vi "tm3samp_framerate_wVision.vi"() -> ()   [LabVIEW 2012]
panel:
  out "Display":T1(plugin-control)
  out "Camera Serial":string
  out "Camera Version":string
  out "Camera Model":string
  out "SMD":dbl
  in  "Scan Mode":dbl min=0.0 max=0.0
  in  "Exposure":dbl min=0.003001263157894737 max=10.0 step=9.74436090225564e-06
  out "EXP":dbl
  out "SVW":i32
  out "SHW":i32
  out "SVO":i32
  out "SHO":i32
  in  "V Width":i32 min=4 max=2048 step=4
  in  "V Offset":i32 min=0 max=0 step=4
  in  "H Width":i32 min=4 max=2048 step=4
  in  "H Offset":i32 min=0 max=0 step=4
  in  "Binning":u16(ring) items=["1x1"=1, "2x2"=2, "4x4"=4]
  out "Elapsed Time":u32
  out "Total Frames":i32
  in  "Display":bool=TRUE
  out "Frames Per Second":dbl
  out "error out":errorcluster
  in  "stop":bool
  # "This example displays the frame rate\nof the camera.  Changing the resolution\nof the camera or displaying the images\nwill affect the frame rate."
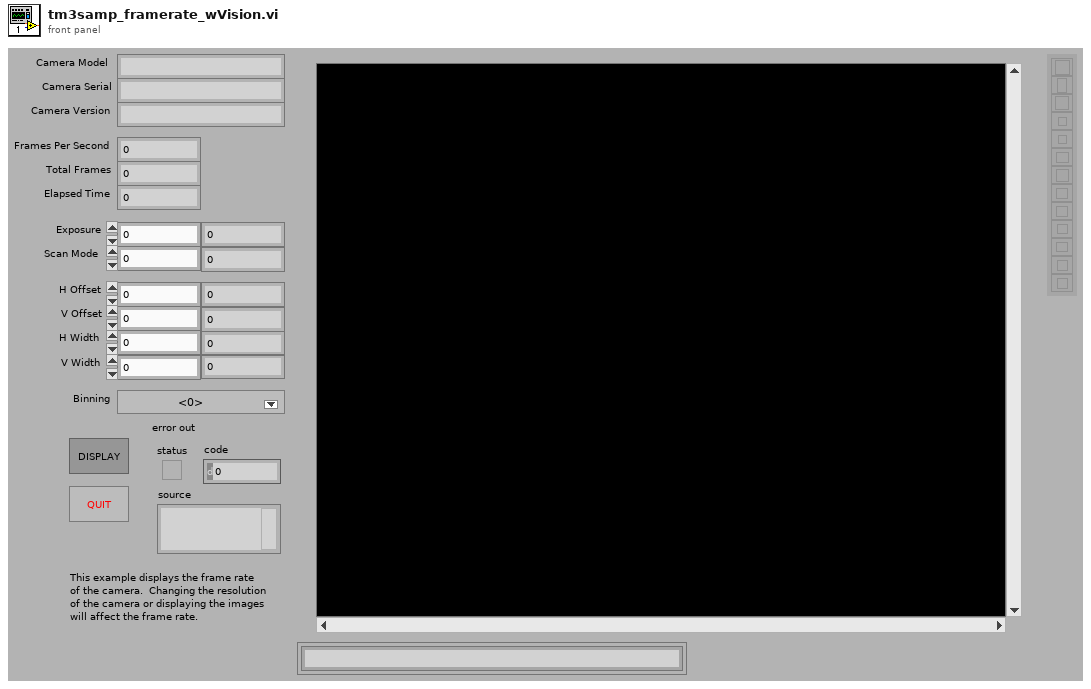
[diagram p1: front panel]
types:
  T1 = typedef "IMAQ Image.ctl" = refnum<image>
  T2 = typedef "Image Type" = u32
  T3 = cluster{"Value":i32, "Minimum":i32, "Maximum":i32, "Increment":i32}
  T4 = cluster{"width":u32, "height":u32, "datatype":u32}
  T5 = cluster{"H Offset":i32, "V Offset":i32, "H Width":i32, "V Width":i32}
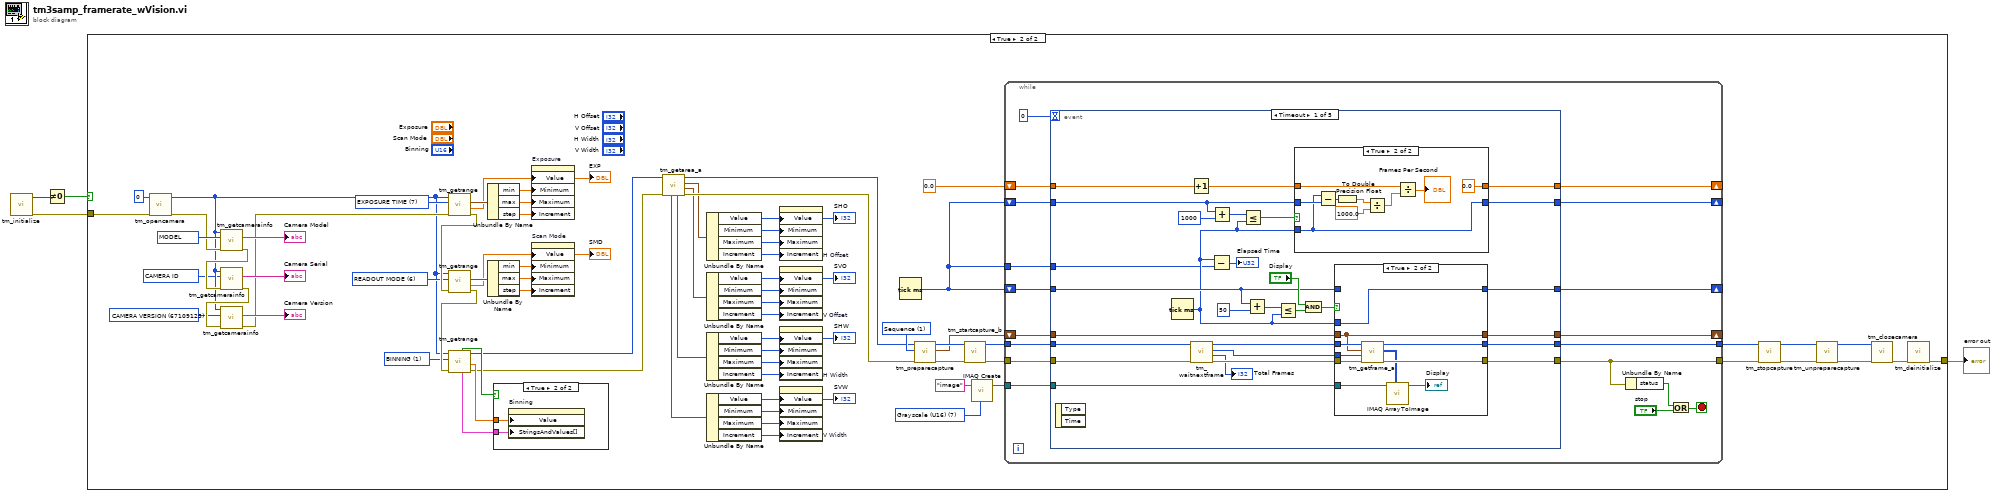
[diagram p0: block diagram]
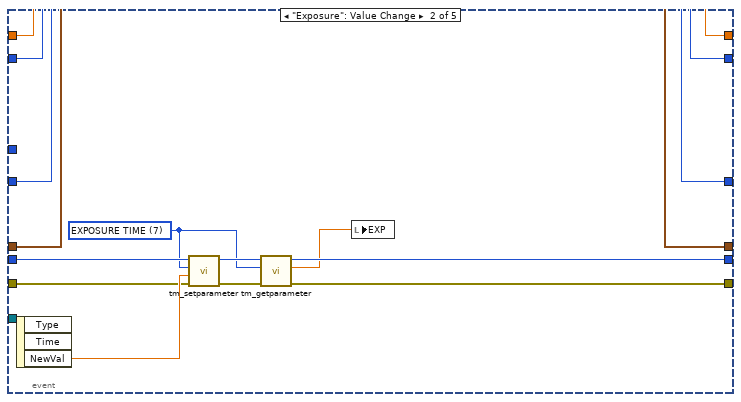
[diagram p6: hidden frame]
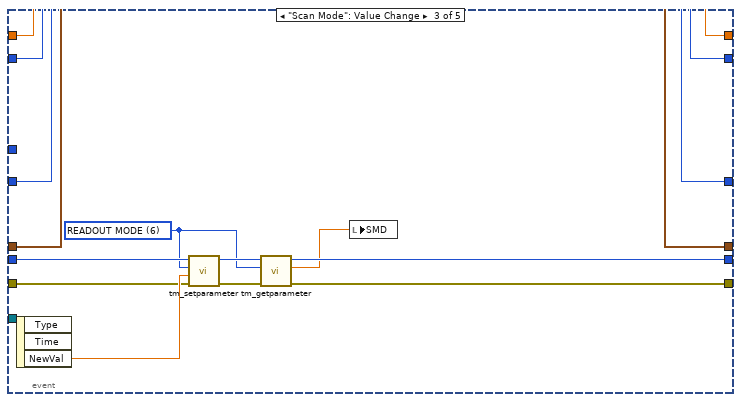
[diagram p7: hidden frame]
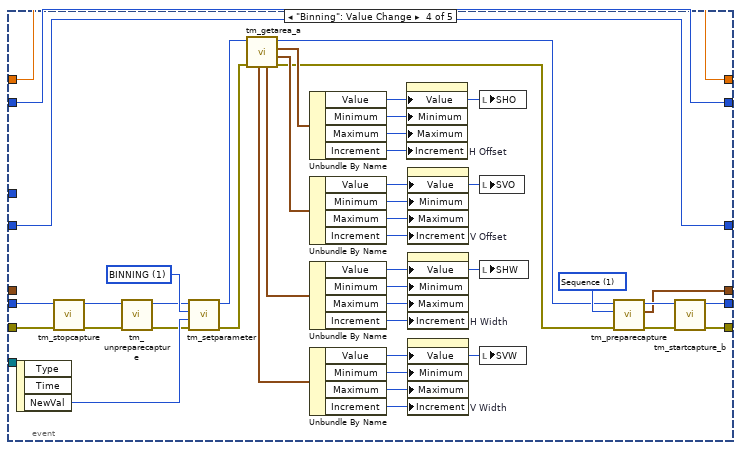
[diagram p8: hidden frame]
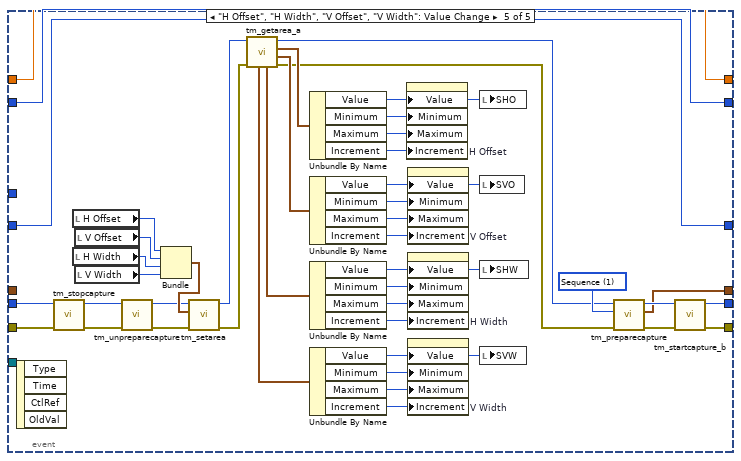
[diagram p9: hidden frame]
diagram:
  n1 = call <userlib>:"tm_initialize.vi"() -> ("error out"=w2:errorcluster, "Number Of Cameras"=w1:u32)  [unwired: 10 in]
  n2 = Not Equal To 0?(x=w1) -> (x != 0?=w4:bool)
  n3 = case shown="True" w4 {
    tunnel: [w5 w76] -> w3
    tunnel: w2 -> [w5 w79]
    frame False {
    }
    frame True {
      w6 = T2 7 items=["Grayscale (U8)", "Grayscale (I16)", "Grayscale (SGL)", "Complex (CSG)", "RGB (U32)", "HSL (U32)", "RGB (U64)", "Grayscale (U16)"] ("Image Type")
      w20 = u32 67109122 items=["BUS"=67109121, "CAMERA ID"=67109122, "VENDOR"=67109123, "MODEL"=67109124, "CAMERA VERSION"=67109125, "DRIVER VERSION"=67109126, "MODULE VERSIOIN"=67109127, "DCAMAPI VERSION"=67109128] ("Info ID")
      w27 = u32 67109125 items=["BUS"=67109121, "CAMERA"=67109122, "VENDOR"=67109123, "MODEL"=67109124, "CAMERA VERSION"=67109125, "DRIVER VERSION"=67109126, "MODULE VERSIOIN"=67109127, "DCAMAPI VERSION"=67109128] ("Info ID")
      w30 = u32 67109124 items=["BUS"=67109121, "CAMERA"=67109122, "VENDOR"=67109123, "MODEL"=67109124, "CAMERA VERSION"=67109125, "DRIVER VERSION"=67109126, "MODULE VERSIOIN"=67109127, "DCAMAPI VERSION"=67109128] ("Info ID")
      w62 = 1 items=["BINNING"=1, "BITS PER CHANNEL"=2, "ACTIVE VIEW INDEX"=3, "CCD MODE"=4, "SENSOR MODE"=5, "READOUT MODE"=6, "EXPOSURE TIME"=7, "CONTRAST GAIN"=8, "CONTRAST OFFSET"=9, "LIGHT MODE"=10, "SENSITIVITY"=11, "WHITE BALANCE"=12, "PHOTON IMAGING MODE"=13, "HIGH DYNAMIC RANGE MODE"=14, "TRIGGER SOURCE"=15, "TRIGGER ACTIVE"=16, "TRIGGER MODE"=17, "TRIGGER POLARITY"=18, "TRIGGER GLOBAL EXPOSURE"=19, "FIRST TRIGGER BEHAVIOR"=20, "TRIGGER TIMES"=21, "OUTPUT TRIGGER POLARITY"=22, "OUTPUT TRIGGER DELAY"=23, "OUTPUT TRIGGER PERIOD"=24, "TEMPERATURE"=25, "TEMPERATURE TARGET"=26, "SENSOR COOLER FAN"=27, "MECHANICAL SHUTTER"=28, "BACK FOCUS POSITION"=29, "FRAMEBUNDLE MODE"=30, "FRAMEBUNDLE NUMBER"=31] ("Parameter")
      w64 = 6 items=["BINNING"=1, "BITS PER CHANNEL"=2, "ACTIVE VIEW INDEX"=3, "CCD MODE"=4, "SENSOR MODE"=5, "READOUT MODE"=6, "EXPOSURE TIME"=7, "CONTRAST GAIN"=8, "CONTRAST OFFSET"=9, "LIGHT MODE"=10, "SENSITIVITY"=11, "WHITE BALANCE"=12, "PHOTON IMAGING MODE"=13, "HIGH DYNAMIC RANGE MODE"=14, "TRIGGER SOURCE"=15, "TRIGGER ACTIVE"=16, "TRIGGER MODE"=17, "TRIGGER POLARITY"=18, "TRIGGER GLOBAL EXPOSURE"=19, "FIRST TRIGGER BEHAVIOR"=20, "TRIGGER TIMES"=21, "OUTPUT TRIGGER POLARITY"=22, "OUTPUT TRIGGER DELAY"=23, "OUTPUT TRIGGER PERIOD"=24, "TEMPERATURE"=25, "TEMPERATURE TARGET"=26, "SENSOR COOLER FAN"=27, "MECHANICAL SHUTTER"=28, "BACK FOCUS POSITION"=29, "FRAMEBUNDLE MODE"=30, "FRAMEBUNDLE NUMBER"=31] ("Parameter")
      w67 = 7 items=["BINNING"=1, "BITS PER CHANNEL"=2, "ACTIVE VIEW INDEX"=3, "CCD MODE"=4, "SENSOR MODE"=5, "READOUT MODE"=6, "EXPOSURE TIME"=7, "CONTRAST GAIN"=8, "CONTRAST OFFSET"=9, "LIGHT MODE"=10, "SENSITIVITY"=11, "WHITE BALANCE"=12, "PHOTON IMAGING MODE"=13, "HIGH DYNAMIC RANGE MODE"=14, "TRIGGER SOURCE"=15, "TRIGGER ACTIVE"=16, "TRIGGER MODE"=17, "TRIGGER POLARITY"=18, "TRIGGER GLOBAL EXPOSURE"=19, "FIRST TRIGGER BEHAVIOR"=20, "TRIGGER TIMES"=21, "OUTPUT TRIGGER POLARITY"=22, "OUTPUT TRIGGER DELAY"=23, "OUTPUT TRIGGER PERIOD"=24, "TEMPERATURE"=25, "TEMPERATURE TARGET"=26, "SENSOR COOLER FAN"=27, "MECHANICAL SHUTTER"=28, "BACK FOCUS POSITION"=29, "FRAMEBUNDLE MODE"=30, "FRAMEBUNDLE NUMBER"=31] ("Parameter")
      w74 = 1 items=["Snap", "Sequence"] ("Capture mode")
      n4 = call <userlib>:"tm_opencamera.vi"("error in (no error)"=w79, "Camera Index"=u32 0) -> ("error out"=w23:errorcluster, "Handle out"=w21:u32)  [unwired: 8 in]
      n5 = call <userlib>:"tm_getcamerainfo.vi"("error in (no error)"=w23, "Info ID"=w30, "Handle in"=w21) -> ("error out"=w29:errorcluster, "String"=→"Camera Model":string)  [unwired: 6 in, 1 out]
      n6 = call <userlib>:"tm_getcamerainfo.vi"("error in (no error)"=w29, "Info ID"=w20, "Handle in"=w21) -> ("error out"=w28:errorcluster, "String"=→"Camera Serial":string)  [unwired: 6 in, 1 out]
      n7 = call <userlib>:"tm_getcamerainfo.vi"("error in (no error)"=w28, "Info ID"=w27, "Handle in"=w21) -> ("error out"=w22:errorcluster, "String"=→"Camera Version":string)  [unwired: 6 in, 1 out]
      n8 = call <userlib>:"tm_getrange.vi"("error in (no error)"=w22, "Parameter"=w67, "Handle in"=w21) -> ("error out"=w65:errorcluster, "default"=w58:dbl, "Range"=w66:cluster{"min":dbl, "max":dbl, "step":dbl})  [unwired: 2 in, 4 out]
      "EXP" <- w58
      n9 = call <userlib>:"tm_getrange.vi"("error in (no error)"=w65, "Parameter"=w64, "Handle in"=w21) -> ("error out"=w63:errorcluster, "default"=w53:dbl, "Range"=w57:cluster{"min":dbl, "max":dbl, "step":dbl})  [unwired: 2 in, 4 out]
      "SMD" <- w53
      n10 = call <userlib>:"tm_getrange.vi"("error in (no error)"=w63, "Parameter"=w62, "Handle in"=w21) -> ("error out"=w48:errorcluster, "default"=w50:dbl, "Handle out"=w49:u32, "Value Names"=w51:cluster{"Name":string, "Value":dbl}[], "Writable"=w52:bool)  [unwired: 2 in, 2 out]
      n11 = Unbundle By Name(w66) -> ("min"=w61:dbl, "max"=w60:dbl, "step"=w59:dbl)
      n12 = Unbundle By Name(w57) -> ("min"=w56:dbl, "max"=w55:dbl, "step"=w54:dbl)
      n13 = case shown="True" w52 {
        tunnel: w51 -> [_ w81]
        tunnel: w50 -> [_ w80]
        frame False {
        }
        frame True {
          n14 = property on="Binning" class="Ring (strict)"("Value"=w80, "StringsAndValues[]"=w81) -> ()  [unwired: 2 in, 2 out]
        }
      }
      n15 = property on="Exposure" class="DigNum (strict)"("Value"=w58, "Minimum"=w61, "Maximum"=w60, "Increment"=w59) -> ()  [unwired: 2 in, 2 out]
      n16 = property on="Scan Mode" class="DigNum (strict)"("Value"=w53, "Minimum"=w56, "Maximum"=w55, "Increment"=w54) -> ()  [unwired: 2 in, 2 out]
      n17 = call <userlib>:"tm_getarea_a.vi"("error in (no error)"=w48, "Handle in"=w49) -> ("error out"=w46:errorcluster, "V Offset"=w45:T3, "H Offset"=w13:T3, "Handle out"=w47:u32, "H Width"=w44:T3, "V Width"=w43:T3)  [unwired: 4 in]
      n18 = Unbundle By Name(w13) -> ("Value"=w12:i32, "Minimum"=w11:i32, "Maximum"=w10:i32, "Increment"=w9:i32)
      "SHO" <- w12
      n19 = Unbundle By Name(w45) -> ("Value"=w33:i32, "Minimum"=w42:i32, "Maximum"=w41:i32, "Increment"=w40:i32)
      "SVO" <- w33
      n20 = Unbundle By Name(w44) -> ("Value"=w32:i32, "Minimum"=w39:i32, "Maximum"=w38:i32, "Increment"=w37:i32)
      "SHW" <- w32
      n21 = Unbundle By Name(w43) -> ("Value"=w31:i32, "Minimum"=w36:i32, "Maximum"=w35:i32, "Increment"=w34:i32)
      "SVW" <- w31
      n22 = property on="H Offset" class="DigNum (strict)"("Value"=w12, "Minimum"=w11, "Maximum"=w10, "Increment"=w9) -> ()  [unwired: 2 in, 2 out]
      n23 = property on="V Offset" class="DigNum (strict)"("Value"=w33, "Minimum"=w42, "Maximum"=w41, "Increment"=w40) -> ()  [unwired: 2 in, 2 out]
      n24 = property on="H Width" class="DigNum (strict)"("Value"=w32, "Minimum"=w39, "Maximum"=w38, "Increment"=w37) -> ()  [unwired: 2 in, 2 out]
      n25 = property on="V Width" class="DigNum (strict)"("Value"=w31, "Minimum"=w36, "Maximum"=w35, "Increment"=w34) -> ()  [unwired: 2 in, 2 out]
      n26 = Tick Count (ms)() -> (millisecond timer value=w68:u32)
      n27 = call <userlib>:"tm_preparecapture.vi"("error in (no error)"=w46, "Capture mode"=w74, "Handle in"=w47) -> ("error out"=w72:errorcluster, "Buffer"=w69:T4, "Handle out"=w73:u32)  [unwired: 5 in, 1 out]
      n28 = call <userlib>:"tm_startcapture_b.vi"("error in (no error)"=w72, "Handle in"=w73) -> ("error out"=w71:errorcluster, "Handle out"=w70:u32)  [unwired: 8 in]
      n29 = call "IMAQ Create"("Image Name"="image", "Image Type"=w6) -> ("New Image"=w7:T1)  [unwired: 3 in, 1 out]
      n30 = while {
        tunnel: w71 -> [w87]
        tunnel: [w85] -> w19
        tunnel: [w84] -> w18
        shift-right: [w94] -> _
        shift-left: w68 -> [w92]
        shift-right: [w95] -> _
        shift-left: 0.0 -> [w93]
        shift-right: [w86] -> _
        shift-left: w68 -> [w90]
        tunnel: w70 -> [w88]
        tunnel: w68 -> [w91]
        shift-right: [w83] -> _
        shift-left: w69 -> [w89]
        tunnel: w7 -> [w82]
        stop <- w97 stop-if-true
        n31 = event shown="[0] Timeout" {
          selector: _ -> [_ _ _ _ _]
          dyn-events: _ -> [_ _ _ _ _]
          timeout: 0 -> [_ _ _ _ _]
          tunnel: [w108 w163 w176 w210 w256] -> w95
          tunnel: [w107 w164 w177 w211 w257] -> w94
          tunnel: w93 -> [w109 w163 w176 w210 w256]
          tunnel: w92 -> [w111 w164 w177 w211 w257]
          tunnel: w91 -> [w103 _ _ _ _]
          tunnel: w90 -> [w112 w166 w179 w220 w264]
          tunnel: w89 -> [w102 w155 w168 _ _]
          tunnel: w88 -> [w114 w161 w174 w185 w226]
          tunnel: w87 -> [w113 w162 w175 w184 w225]
          tunnel: [w106 w166 w179 w220 w264] -> w86
          tunnel: [w105 w157 w170 w214 w259] -> w85
          tunnel: [w104 w156 w169 w215 w260] -> w84
          tunnel: [w101 w155 w168 w213 w258] -> w83
          tunnel: w82 -> [w100 _ _ _ _]
          event Timeout {
            n32 = event-data() -> ()  [unwired: 1 in, 2 out]
            n33 = Tick Count (ms)() -> (millisecond timer value=w110:u32)
            n34 = Increment(x=w109) -> (x+1=w125:dbl)
            n35 = call <userlib>:"tm_waitnextframe.vi"("error in (no error)"=w113, "Handle in"=w114) -> ("error out"=w119:errorcluster, "Frame Count"=→"Total Frames":i32, "Frame Index"=w118:i32, "Handle out"=w120:u32)  [unwired: 6 in]
            n36 = Subtract(x=w110, y=w103) -> (x-y=→"Elapsed Time":u32)
            n37 = Add(x=w111, y=u32 1000) -> (x+y=w128:u32)
            n38 = Less Or Equal?(x=w128, y=w110) -> (x <= y?=w127:bool)
            n39 = Add(x=w112, y=u32 50) -> (x+y=w124:u32)
            n40 = Less Or Equal?(x=w124, y=w110) -> (x <= y?=w122:bool)
            n41 = case shown="True" w127 {
              tunnel: w111 -> [w144 w147]
              tunnel: [w144 w145] -> w107
              tunnel: w125 -> [w143 w151]
              tunnel: w110 -> [_ w145]
              tunnel: [w143 0.0] -> w108
              frame False {
              }
              frame True {
                n42 = Subtract(x=w145, y=w147) -> (x-y=w146:u32)
                n43 = To Double Precision Float(number=w146) -> (double precision float=w153:dbl)
                n44 = Divide(x=w153, y=1000.0) -> (x/y=w150:dbl)
                n45 = Divide(x=w151, y=w150) -> (x/y=→"Frames Per Second":dbl)
              }
            }
            n46 = And(x="Display", y=w122) -> (x .and. y?=w117:bool)
            n47 = case shown="True" w117 {
              tunnel: w112 -> [w132 _]
              tunnel: w110 -> [_ w142]
              tunnel: [w132 w142] -> w106
              tunnel: w120 -> [w131 w141]
              tunnel: w102 -> [w129 w136]
              tunnel: w119 -> [w130 w140]
              tunnel: [w131 w139] -> w105
              tunnel: [w130 w138] -> w104
              tunnel: w118 -> [_ w137]
              tunnel: [w129 w136] -> w101
              tunnel: w100 -> [_ w134]
              frame False {
              }
              frame True {
                n48 = call <userlib>:"tm_getframe_a.vi"("error in (no error)"=w140, "Frame Index"=w137, "Buffer"=w136, "Handle in"=w141) -> ("error out"=w138:errorcluster, "Data 16"=w135:u16[][], "Handle out"=w139:u32)  [unwired: 3 in, 2 out]
                n49 = call "IMAQ ArrayToImage"("Image Pixels (U16)"=w135, "Image"=w134) -> ("Image Out"=→"Display":T1)  [unwired: 8 in, 1 out]
              }
            }
          }
          event "Exposure": Value Change {
            w158 = 7 items=["BINNING"=1, "BITS PER CHANNEL"=2, "ACTIVE VIEW INDEX"=3, "CCD MODE"=4, "SENSOR MODE"=5, "READOUT MODE"=6, "EXPOSURE TIME"=7, "CONTRAST GAIN"=8, "CONTRAST OFFSET"=9, "LIGHT MODE"=10, "SENSITIVITY"=11, "WHITE BALANCE"=12, "PHOTON IMAGING MODE"=13, "HIGH DYNAMIC RANGE MODE"=14, "TRIGGER SOURCE"=15, "TRIGGER ACTIVE"=16, "TRIGGER MODE"=17, "TRIGGER POLARITY"=18, "TRIGGER GLOBAL EXPOSURE"=19, "FIRST TRIGGER BEHAVIOR"=20, "TRIGGER TIMES"=21, "OUTPUT TRIGGER POLARITY"=22, "OUTPUT TRIGGER DELAY"=23, "OUTPUT TRIGGER PERIOD"=24, "TEMPERATURE"=25, "TEMPERATURE TARGET"=26, "SENSOR COOLER FAN"=27, "MECHANICAL SHUTTER"=28, "BACK FOCUS POSITION"=29, "FRAMEBUNDLE MODE"=30, "FRAMEBUNDLE NUMBER"=31] ("Parameter")
            n50 = event-data() -> ("NewVal"=w165:dbl)  [unwired: 1 in, 2 out]
            n51 = call <userlib>:"tm_setparameter.vi"("error in (no error)"=w162, "Value in"=w165, "Parameter"=w158, "Handle in"=w161) -> ("error out"=w160:errorcluster, "Handle out"=w159:u32)  [unwired: 6 in]
            n52 = call <userlib>:"tm_getparameter.vi"("error in (no error)"=w160, "Parameter"=w158, "Handle in"=w159) -> ("error out"=w156:errorcluster, "Value out"=w154:dbl, "Handle out"=w157:u32)  [unwired: 6 in]
            n53 = local write "EXP"(w154) -> ()
          }
          event "Scan Mode": Value Change {
            w171 = 6 items=["BINNING"=1, "BITS PER CHANNEL"=2, "ACTIVE VIEW INDEX"=3, "CCD MODE"=4, "SENSOR MODE"=5, "READOUT MODE"=6, "EXPOSURE TIME"=7, "CONTRAST GAIN"=8, "CONTRAST OFFSET"=9, "LIGHT MODE"=10, "SENSITIVITY"=11, "WHITE BALANCE"=12, "PHOTON IMAGING MODE"=13, "HIGH DYNAMIC RANGE MODE"=14, "TRIGGER SOURCE"=15, "TRIGGER ACTIVE"=16, "TRIGGER MODE"=17, "TRIGGER POLARITY"=18, "TRIGGER GLOBAL EXPOSURE"=19, "FIRST TRIGGER BEHAVIOR"=20, "TRIGGER TIMES"=21, "OUTPUT TRIGGER POLARITY"=22, "OUTPUT TRIGGER DELAY"=23, "OUTPUT TRIGGER PERIOD"=24, "TEMPERATURE"=25, "TEMPERATURE TARGET"=26, "SENSOR COOLER FAN"=27, "MECHANICAL SHUTTER"=28, "BACK FOCUS POSITION"=29, "FRAMEBUNDLE MODE"=30, "FRAMEBUNDLE NUMBER"=31] ("Parameter")
            n54 = event-data() -> ("NewVal"=w178:dbl)  [unwired: 1 in, 2 out]
            n55 = call <userlib>:"tm_setparameter.vi"("error in (no error)"=w175, "Value in"=w178, "Parameter"=w171, "Handle in"=w174) -> ("error out"=w173:errorcluster, "Handle out"=w172:u32)  [unwired: 6 in]
            n56 = call <userlib>:"tm_getparameter.vi"("error in (no error)"=w173, "Parameter"=w171, "Handle in"=w172) -> ("error out"=w169:errorcluster, "Value out"=w167:dbl, "Handle out"=w170:u32)  [unwired: 6 in]
            n57 = local write "SMD"(w167) -> ()
          }
          event "Binning": Value Change {
            w218 = 1 items=["Snap", "Sequence"] ("Capture mode")
            w219 = 1 items=["BINNING"=1, "BITS PER CHANNEL"=2, "ACTIVE VIEW INDEX"=3, "CCD MODE"=4, "SENSOR MODE"=5, "READOUT MODE"=6, "EXPOSURE TIME"=7, "CONTRAST GAIN"=8, "CONTRAST OFFSET"=9, "LIGHT MODE"=10, "SENSITIVITY"=11, "WHITE BALANCE"=12, "PHOTON IMAGING MODE"=13, "HIGH DYNAMIC RANGE MODE"=14, "TRIGGER SOURCE"=15, "TRIGGER ACTIVE"=16, "TRIGGER MODE"=17, "TRIGGER POLARITY"=18, "TRIGGER GLOBAL EXPOSURE"=19, "FIRST TRIGGER BEHAVIOR"=20, "TRIGGER TIMES"=21, "OUTPUT TRIGGER POLARITY"=22, "OUTPUT TRIGGER DELAY"=23, "OUTPUT TRIGGER PERIOD"=24, "TEMPERATURE"=25, "TEMPERATURE TARGET"=26, "SENSOR COOLER FAN"=27, "MECHANICAL SHUTTER"=28, "BACK FOCUS POSITION"=29, "FRAMEBUNDLE MODE"=30, "FRAMEBUNDLE NUMBER"=31] ("Parameter")
            n58 = event-data() -> ("NewVal"=w212:u16)  [unwired: 1 in, 2 out]
            n59 = call <userlib>:"tm_stopcapture.vi"("error in (no error)"=w184, "Handle in"=w185) -> ("error out"=w180:errorcluster, "Handle out"=w183:u32)  [unwired: 8 in]
            n60 = call <userlib>:"tm_unpreparecapture.vi"("error in (no error)"=w180, "Handle in"=w183) -> ("error out"=w181:errorcluster, "Handle out"=w182:u32)  [unwired: 8 in]
            n61 = call <userlib>:"tm_setparameter.vi"("error in (no error)"=w181, "Value in"=w212, "Parameter"=w219, "Handle in"=w182) -> ("error out"=w204:errorcluster, "Handle out"=w205:u32)  [unwired: 6 in]
            n62 = call <userlib>:"tm_getarea_a.vi"("error in (no error)"=w204, "Handle in"=w205) -> ("error out"=w203:errorcluster, "V Offset"=w207:T3, "H Offset"=w206:T3, "Handle out"=w202:u32, "H Width"=w208:T3, "V Width"=w209:T3)  [unwired: 4 in]
            n63 = Unbundle By Name(w206) -> ("Value"=w198:i32, "Minimum"=w201:i32, "Maximum"=w200:i32, "Increment"=w199:i32)
            n64 = Unbundle By Name(w207) -> ("Value"=w188:i32, "Minimum"=w197:i32, "Maximum"=w196:i32, "Increment"=w195:i32)
            n65 = Unbundle By Name(w208) -> ("Value"=w187:i32, "Minimum"=w194:i32, "Maximum"=w193:i32, "Increment"=w192:i32)
            n66 = Unbundle By Name(w209) -> ("Value"=w186:i32, "Minimum"=w191:i32, "Maximum"=w190:i32, "Increment"=w189:i32)
            n67 = property on="H Offset" class="DigNum (strict)"("Value"=w198, "Minimum"=w201, "Maximum"=w200, "Increment"=w199) -> ()  [unwired: 2 in, 2 out]
            n68 = property on="V Offset" class="DigNum (strict)"("Value"=w188, "Minimum"=w197, "Maximum"=w196, "Increment"=w195) -> ()  [unwired: 2 in, 2 out]
            n69 = property on="H Width" class="DigNum (strict)"("Value"=w187, "Minimum"=w194, "Maximum"=w193, "Increment"=w192) -> ()  [unwired: 2 in, 2 out]
            n70 = property on="V Width" class="DigNum (strict)"("Value"=w186, "Minimum"=w191, "Maximum"=w190, "Increment"=w189) -> ()  [unwired: 2 in, 2 out]
            n71 = local write "SHO"(w198) -> ()
            n72 = local write "SVO"(w188) -> ()
            n73 = local write "SHW"(w187) -> ()
            n74 = local write "SVW"(w186) -> ()
            n75 = call <userlib>:"tm_preparecapture.vi"("error in (no error)"=w203, "Capture mode"=w218, "Handle in"=w202) -> ("error out"=w216:errorcluster, "Buffer"=w213:T4, "Handle out"=w217:u32)  [unwired: 5 in, 1 out]
            n76 = call <userlib>:"tm_startcapture_b.vi"("error in (no error)"=w216, "Handle in"=w217) -> ("error out"=w215:errorcluster, "Handle out"=w214:u32)  [unwired: 8 in]
          }
          event "H Offset", "H Width", "V Offset", "V Width": Value Change {
            w263 = 1 items=["Snap", "Sequence"] ("Capture mode")
            n77 = event-data() -> ()  [unwired: 1 in, 4 out]
            n78 = call <userlib>:"tm_stopcapture.vi"("error in (no error)"=w225, "Handle in"=w226) -> ("error out"=w223:errorcluster, "Handle out"=w224:u32)  [unwired: 8 in]
            n79 = local read "H Offset"() -> (w229:i32)
            n80 = local read "H Width"() -> (w230:i32)
            n81 = local read "V Offset"() -> (w231:i32)
            n82 = local read "V Width"() -> (w228:i32)
            n83 = call <userlib>:"tm_unpreparecapture.vi"("error in (no error)"=w223, "Handle in"=w224) -> ("error out"=w221:errorcluster, "Handle out"=w222:u32)  [unwired: 8 in]
            n84 = Bundle("H Offset"=w229, "V Offset"=w231, "H Width"=w230, "V Width"=w228) -> (w227:T5)  [unwired: 1 in]
            n85 = call <userlib>:"tm_setarea.vi"("error in (no error)"=w221, "Sub Region"=w227, "Handle in"=w222) -> ("error out"=w232:errorcluster, "Handle out"=w233:u32)  [unwired: 7 in]
            n86 = call <userlib>:"tm_getarea_a.vi"("error in (no error)"=w232, "Handle in"=w233) -> ("error out"=w251:errorcluster, "V Offset"=w253:T3, "H Offset"=w252:T3, "Handle out"=w250:u32, "H Width"=w254:T3, "V Width"=w255:T3)  [unwired: 4 in]
            n87 = Unbundle By Name(w252) -> ("Value"=w246:i32, "Minimum"=w249:i32, "Maximum"=w248:i32, "Increment"=w247:i32)
            n88 = Unbundle By Name(w253) -> ("Value"=w236:i32, "Minimum"=w245:i32, "Maximum"=w244:i32, "Increment"=w243:i32)
            n89 = Unbundle By Name(w254) -> ("Value"=w235:i32, "Minimum"=w242:i32, "Maximum"=w241:i32, "Increment"=w240:i32)
            n90 = Unbundle By Name(w255) -> ("Value"=w234:i32, "Minimum"=w239:i32, "Maximum"=w238:i32, "Increment"=w237:i32)
            n91 = property on="H Offset" class="DigNum (strict)"("Value"=w246, "Minimum"=w249, "Maximum"=w248, "Increment"=w247) -> ()  [unwired: 2 in, 2 out]
            n92 = property on="V Offset" class="DigNum (strict)"("Value"=w236, "Minimum"=w245, "Maximum"=w244, "Increment"=w243) -> ()  [unwired: 2 in, 2 out]
            n93 = property on="H Width" class="DigNum (strict)"("Value"=w235, "Minimum"=w242, "Maximum"=w241, "Increment"=w240) -> ()  [unwired: 2 in, 2 out]
            n94 = property on="V Width" class="DigNum (strict)"("Value"=w234, "Minimum"=w239, "Maximum"=w238, "Increment"=w237) -> ()  [unwired: 2 in, 2 out]
            n95 = local write "SHO"(w246) -> ()
            n96 = local write "SVO"(w236) -> ()
            n97 = local write "SHW"(w235) -> ()
            n98 = local write "SVW"(w234) -> ()
            n99 = call <userlib>:"tm_preparecapture.vi"("error in (no error)"=w251, "Capture mode"=w263, "Handle in"=w250) -> ("error out"=w261:errorcluster, "Buffer"=w258:T4, "Handle out"=w262:u32)  [unwired: 5 in, 1 out]
            n100 = call <userlib>:"tm_startcapture_b.vi"("error in (no error)"=w261, "Handle in"=w262) -> ("error out"=w260:errorcluster, "Handle out"=w259:u32)  [unwired: 8 in]
          }
        }
        n101 = Unbundle By Name(w84) -> ("status"=w98:bool)
        n102 = Or(x=w98, y="stop") -> (x .or. y?=w97:bool)
      }
      n103 = call <userlib>:"tm_stopcapture.vi"("error in (no error)"=w18, "Handle in"=w19) -> ("error out"=w15:errorcluster, "Handle out"=w16:u32)  [unwired: 8 in]
      n104 = call <userlib>:"tm_unpreparecapture.vi"("error in (no error)"=w15, "Handle in"=w16) -> ("error out"=w14:errorcluster, "Handle out"=w17:u32)  [unwired: 8 in]
      n105 = call <userlib>:"tm_closecamera.vi"("error in (no error)"=w14, "Handle in"=w17) -> ("error out"=w77:errorcluster)  [unwired: 9 in]
      n106 = call <userlib>:"tm_deinitialize.vi"("error in (no error)"=w77) -> ("error out"=w76:errorcluster)  [unwired: 10 in]
    }
  }
  "error out" <- w3
